vi "Read Command Settings.vi"(8 "error in (no error)":errorcluster, 11 "WriteCommand in":refnum<class "WriteCommand.lvclass">) -> (0 "error out":errorcluster, 2 "Command Settings":refnum<class "CommandSetting.lvclass">[](array[class]), 3 "WriteCommand out":refnum<class "WriteCommand.lvclass">)   [LabVIEW 2023, in "HAF.lvlib" / "WriteCommand.lvclass"]
doc: "Returns the current Command Settings."
uses:
  WriteCommand.lvclass
  CommandSetting/CommandSetting.lvclass
  WriteCommand.lvclass/WriteCommand.ctl
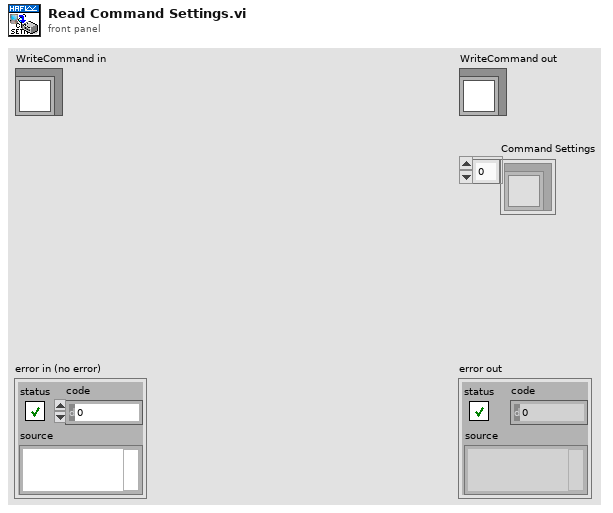
[diagram p1: front panel]
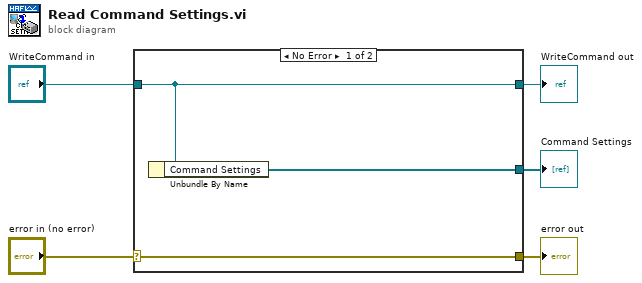
[diagram p0: block diagram]
diagram:
  n1 = case shown="No Error" "error in (no error)" {
    selector: "error in (no error)" -> [w8 w9]
    tunnel: [w8 w9] -> w4
    tunnel: [w7 w10] -> w2
    tunnel: "WriteCommand in" -> [w7 w10]
    tunnel: [w6 _] -> w1
    frame No Error {
      n2 = Unbundle By Name(w7) -> ("Command Settings"=w6:refnum<class "CommandSetting.lvclass">[])
    }
    frame Error {
    }
  }
  "error out" <- w4
  "WriteCommand out" <- w2
  "Command Settings" <- w1
